vi "NEVSTOP-3rdParty-Dependencies_Post-Install Custom Action.vi"(10 "Variant":variant) -> (0 "error out":errorcluster)   [LabVIEW 2014]
uses:
  <vilib>/Palette API/Palette Menu/Public Type Define/Palette type.ctl
  <vilib>/Palette API/Palette Menu/Palette Menu.lvlib
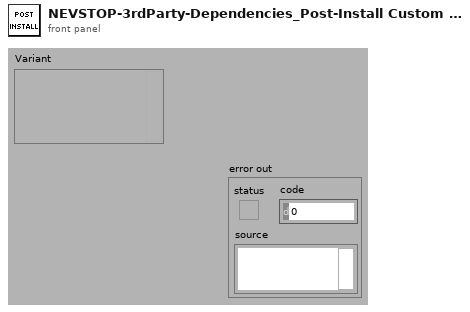
[diagram p1: front panel]
types:
  T1 = typedef "Palette Menu.lvlib/Palette type.ctl" = i32
  T2 = typedef "Palette Menu.lvlib/Palette Data.ctl" = cluster{"display name":string, "view format":T3, "palette width":i16, "items":T4, "256 color icon":picture, "B&W color icon":picture, "help information":T6, "palette description":string, "synchronize information":T7}
  T3 = typedef "Palette Menu.lvlib/View Format.ctl" = u16
  T4 = typedef "Palette Menu.lvlib/Items.ctl" = T5[]
  T5 = typedef "Palette Menu.lvlib/Item.ctl" = cluster{"item path":path, "library path (.lvlib)":path, "use default lvlib palette":bool, "short name":string, "place VI contents":bool, "hide synchronized item":bool, "reserve spot for synch item":bool, "configure when placing VI contents":bool}
  T6 = typedef "Palette Menu.lvlib/Help Info.ctl" = cluster{"help tag":string, "help file path ":path}
  T7 = typedef "Palette Menu.lvlib/Synchronize Info.ctl" = cluster{"synchronize with directory":bool, "synchronize directory path":path}
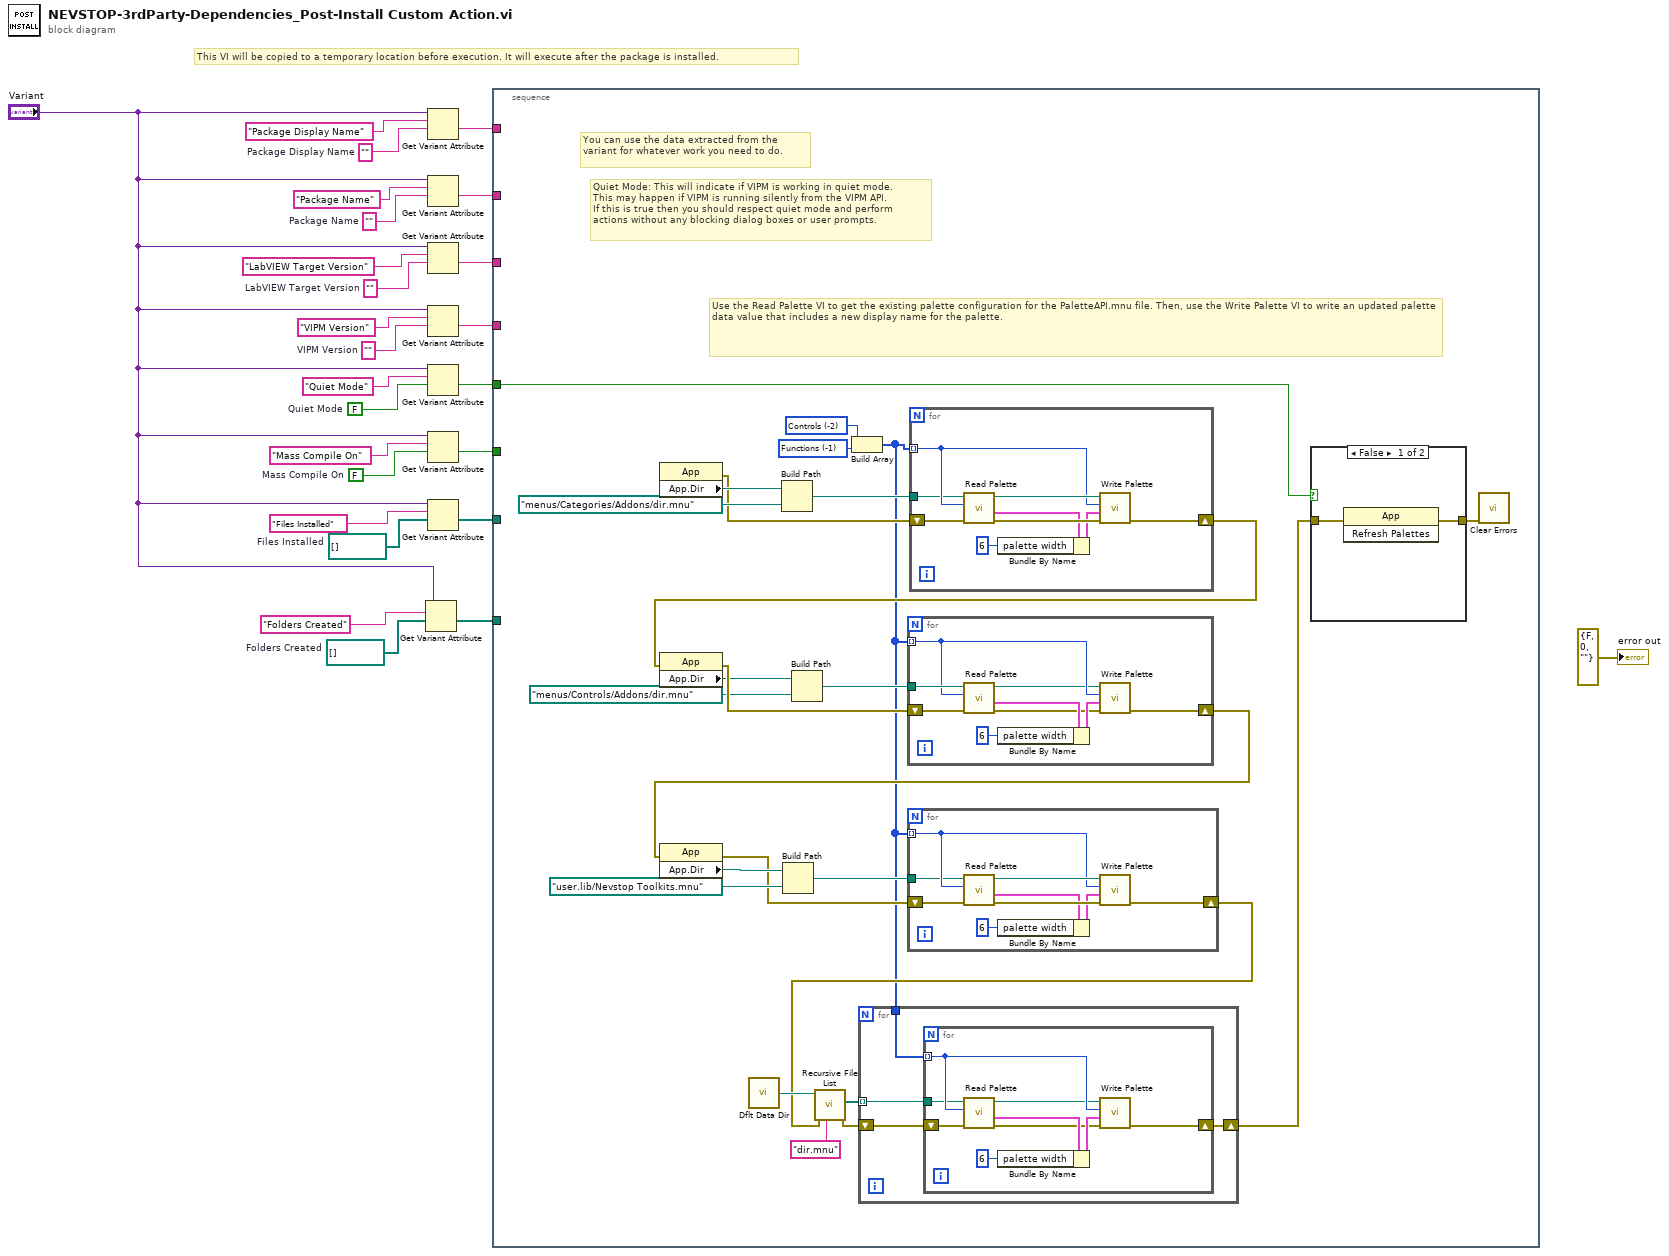
[diagram p0: block diagram]
diagram:
  w1 = path[] []  # Folders Created
  w2 = path[] []  # Files Installed
  w8 = FALSE  # Mass Compile On
  w9 = ""  # Package Display Name
  w16 = FALSE  # Quiet Mode
  w19 = ""  # VIPM Version
  w21 = ""  # LabVIEW Target Version
  w23 = ""  # Package Name
  # "This VI will be copied to a temporary location before execution. It will execute after the package is installed."
  n1 = Get Variant Attribute(Variant="Variant", name="Folders Created", default value (empty Variant)=w1) -> (value=w6:path[])  [unwired: 1 in, 3 out]
  n2 = Get Variant Attribute(Variant="Variant", name="Package Display Name", default value (empty Variant)=w9) -> (value=w15:string)  [unwired: 1 in, 3 out]
  n3 = Get Variant Attribute(Variant="Variant", name="Package Name", default value (empty Variant)=w23) -> (value=w14:string)  [unwired: 1 in, 3 out]
  n4 = Get Variant Attribute(Variant="Variant", name="LabVIEW Target Version", default value (empty Variant)=w21) -> (value=w13:string)  [unwired: 1 in, 3 out]
  n5 = Get Variant Attribute(Variant="Variant", name="VIPM Version", default value (empty Variant)=w19) -> (value=w12:string)  [unwired: 1 in, 3 out]
  n6 = Get Variant Attribute(Variant="Variant", name="Quiet Mode", default value (empty Variant)=w16) -> (value=w11:bool)  [unwired: 1 in, 3 out]
  n7 = Get Variant Attribute(Variant="Variant", name="Mass Compile On", default value (empty Variant)=w8) -> (value=w10:bool)  [unwired: 1 in, 3 out]
  n8 = Get Variant Attribute(Variant="Variant", name="Files Installed", default value (empty Variant)=w2) -> (value=w5:path[])  [unwired: 1 in, 3 out]
  n9 = stacked-sequence {
    tunnel: w15 -> [_]
    tunnel: w14 -> [_]
    tunnel: w13 -> [_]
    tunnel: w12 -> [_]
    tunnel: w11 -> [w40]
    tunnel: w10 -> [_]
    tunnel: w5 -> [_]
    tunnel: w6 -> [_]
    frame #0 {
      w28 = T1 -2 items=["Functions"=-1, "Controls"=-2] ("palette type")
      w50 = T1 -1 items=["Functions"=-1, "Controls"=-2] ("palette type")
      # "Use the Read Palette VI to get the existing palette configuration for the PaletteAPI.mnu file. Then, use the Write Palette VI to write an updated palette data value that includes a new display name for the palette."
      # "Quiet Mode: This will indicate if VIPM is working in quiet mode.\nThis may happen if VIPM is running silently from the VIPM API.\nIf this is true then you should respect quiet mode and perform\nactions without any blocking dialog boxes or user prompts."
      # "You can use the data extracted from the variant for whatever work you need to do."
      n10 = property class="App"() -> (error out=w46:errorcluster, "App.Dir"=w49:path)  [unwired: 2 in, 1 out]
      n11 = call <vilib>:"Dflt Data Dir.vi"() -> ("App:Default Data Directory"=w39:path)
      n12 = Build Path(base path=w49, name or relative path=path "menus/Categories/Addons/dir.mnu") -> (appended path=w48:path)
      n13 = Build Array(w28, w50) -> (w27:T1[])
      n14 = for {
        tunnel: w27 -> [w74] mode=indexing
        tunnel: w48 -> [w73]
        shift-right: [w70] -> w41
        shift-left: w46 -> [w72]
        n15 = call <vilib>:"Read Palette.vi"("error in (no error)"=w72, "palette type"=w74, "palette path"=w73) -> ("error out"=w78:errorcluster, "palette data"=w77:T2, "duplicate palette path"=w75:path)  [unwired: 1 in, 5 out]
        n16 = Bundle By Name(cluster=w77, "palette width"=i16 6) -> (w76:T2)
        n17 = call <vilib>:"Write Palette.vi"("error in (no error)"=w78, "palette data"=w76, "palette type"=w74, "palette path"=w75) -> ("error out"=w70:errorcluster)  [unwired: 1 in, 6 out]
      }
      n18 = property class="App"(error in=w41) -> (error out=w45:errorcluster, "App.Dir"=w42:path)  [unwired: 1 in, 1 out]
      n19 = Build Path(base path=w42, name or relative path=path "menus/Controls/Addons/dir.mnu") -> (appended path=w43:path)
      n20 = for {
        tunnel: w43 -> [w67]
        tunnel: w27 -> [w66] mode=indexing
        shift-right: [w61] -> w30
        shift-left: w45 -> [w68]
        n21 = call <vilib>:"Read Palette.vi"("error in (no error)"=w68, "palette type"=w66, "palette path"=w67) -> ("error out"=w62:errorcluster, "palette data"=w63:T2, "duplicate palette path"=w65:path)  [unwired: 1 in, 5 out]
        n22 = Bundle By Name(cluster=w63, "palette width"=i16 6) -> (w64:T2)
        n23 = call <vilib>:"Write Palette.vi"("error in (no error)"=w62, "palette data"=w64, "palette type"=w66, "palette path"=w65) -> ("error out"=w61:errorcluster)  [unwired: 1 in, 6 out]
      }
      n24 = property class="App"(error in=w30) -> (error out=w31:errorcluster, "App.Dir"=w34:path)  [unwired: 1 in, 1 out]
      n25 = Build Path(base path=w34, name or relative path=path "user.lib/Nevstop Toolkits.mnu") -> (appended path=w33:path)
      n26 = for {
        tunnel: w27 -> [w56] mode=indexing
        tunnel: w33 -> [w55]
        shift-right: [w52] -> w29
        shift-left: w31 -> [w54]
        n27 = call <vilib>:"Read Palette.vi"("error in (no error)"=w54, "palette type"=w56, "palette path"=w55) -> ("error out"=w60:errorcluster, "palette data"=w59:T2, "duplicate palette path"=w57:path)  [unwired: 1 in, 5 out]
        n28 = Bundle By Name(cluster=w59, "palette width"=i16 6) -> (w58:T2)
        n29 = call <vilib>:"Write Palette.vi"("error in (no error)"=w60, "palette data"=w58, "palette type"=w56, "palette path"=w57) -> ("error out"=w52:errorcluster)  [unwired: 1 in, 6 out]
      }
      n30 = call <vilib>:"Recursive File List.vi"("pattern"="dir.mnu", "error in (no error)"=w29, "Folder Path"=w39) -> ("error out"=w36:errorcluster, "All Files in Dir"=w37:path[])  [unwired: 4 in, 3 out]
      n31 = for {
        tunnel: w37 -> [w82] mode=indexing
        shift-right: [w80] -> w35
        shift-left: w36 -> [w81]
        tunnel: w27 -> [w79]
        n32 = for {
          tunnel: w79 -> [w90] mode=indexing
          tunnel: w82 -> [w85]
          shift-right: [w83] -> w80
          shift-left: w81 -> [w84]
          n33 = call <vilib>:"Read Palette.vi"("error in (no error)"=w84, "palette type"=w90, "palette path"=w85) -> ("error out"=w86:errorcluster, "palette data"=w87:T2, "duplicate palette path"=w89:path)  [unwired: 1 in, 5 out]
          n34 = Bundle By Name(cluster=w87, "palette width"=i16 6) -> (w88:T2)
          n35 = call <vilib>:"Write Palette.vi"("error in (no error)"=w86, "palette data"=w88, "palette type"=w90, "palette path"=w89) -> ("error out"=w83:errorcluster)  [unwired: 1 in, 6 out]
        }
      }
      n36 = case shown="False" w40 {
        tunnel: [w93 w94] -> w51
        tunnel: w35 -> [w92 w94]
        frame False {
          n37 = invoke class="App" method="Refresh Palettes"(error in=w92) -> (error out=w93:errorcluster)  [unwired: 2 in, 2 out]
        }
        frame True {
        }
      }
      n38 = call <vilib>:"Clear Errors.vi"("error in (no error)"=w51) -> ()  [unwired: 6 in, 1 out]
    }
  }
  "error out" <- errorcluster {"status"=FALSE, "code"=0, "source"=""} ("error out")
